vi "f_main_2014.vi"() -> ()   [LabVIEW 2014]
uses:
  <vilib>/Platform/TimedLoop/XDataNode/timing_clust.ctl
  <vilib>/Platform/TimedLoop/XDataNode/nitl_modes.ctl
  <vilib>/Platform/TimedLoop/XDataNode/wakeup.ctl
  <vilib>/rvi/Emulation/niFpgaGetClockAttributes.vi
  <vilib>/rvi/Emulation/niFpgaSctlEmulationGetInTimedLoop.vi
  <vilib>/rvi/Emulation/niFpgaEmulationReportErrorSimple.vi
  <vilib>/rvi/Emulation/niFpgaProcessEmulError.vi
  <vilib>/rvi/eio/common/nirviEmuTemplateMethod_errors.vi
  <vilib>/rvi/occurrence/nirviWaitOnOccurrenceBase.vi
  <vilib>/rvi/Emulation/niFpgaCriticalErrorInLSC.vi
  Instance           4 21Saved   f_main(DMA)85 .vi
  Instance           5 21Saved   f_main(DMA)85 .vi
  Instance           6 21Saved   f_main(DMA)85 .vi
  <vilib>/rvi/Memory/Memory_Emulation/nirvimemoryFastEmulation.vi
  <vilib>/rvi/Memory/Memory_Emulation/nirvimemoryEmulation.vi
  <vilib>/rvi/Emulation/niFpgaEmulationIsFPGAContextNoSignature.vi
  <vilib>/rvi/DataTransferAndStorage/Container/Common/niFpgaContainerGetUniqueNameForEmu.vi
  <vilib>/rvi/errors/nirviReportUnexpectedCaseInternalError (U32).vi
  <vilib>/rvi/interface/RandomDataEmulation/niFpgaRandomDataHandleErrors.vi
  Instance           2 21Saved   f_main(DMA)85 .vi
  Instance           3 21Saved   f_main(DMA)85 .vi
  <vilib>/eio/EIONode/EIONode.xnode
  <vilib>/Platform/TimedLoop/XDataNode/XDataNode.xnode
  <vilib>/rvi/DataTransferAndStorage/Container/XNode/niFpgaContainer.xnode
  <vilib>/rvi/interface/RandomDataEmulation/nirviRandomDataFpgaReadWriteTemplate.vi
  <vilib>/Platform/TimedLoop/XDataNode/XDNodeRunTimeDep.lvlib
panel:
  out "SampleTrigger3":u32
  out "SampleTrigger2":u32
  out "SampleTrigger1":u32
  out "SampleTrigger0":u32
  out "C3DIGIN":bool
  out "C2DIGIN":bool
  out "C0DIGIN":bool
  out "C1DIGIN":bool
  out "C3ADDREnable":bool
  out "C3Auswahl":bool
  out "C3ADDR3":bool
  out "C3ADDR2":bool
  out "C3ADDR1":bool
  out "C3ADDR0":bool
  out "C2ADDREnable":bool
  out "C2Auswahl":bool
  out "C2ADDR3":bool
  out "C2ADDR2":bool
  out "C2ADDR1":bool
  out "C2ADDR0":bool
  out "C1ADDREnable":bool
  out "C1Auswahl":bool
  out "C1ADDR3":bool
  out "C1ADDR2":bool
  out "C1ADDR1":bool
  out "C1ADDR0":bool
  in  "Test":bool
  in  "Timeout(in Ticks)":u32=4294967295
  out "cancel":bool
  out "Timeout":bool
  out "Sprung1":bool
  out "Sprung0":bool
  out "Fifo-Fehler":bool
  out "in\nReady":bool
  out "ScanID":u32
  in  "ADCRead":bool
  in  "read_count":u32
  out "C0ADDREnable":bool
  out "C0Auswahl":bool
  out "C0ADDR3":bool
  out "C0ADDR2":bool
  out "C0ADDR1":bool
  out "C0ADDR0":bool
  in  "SPIWrite":bool
  in  "Serial Data Out":bool[](array[boolean])=[FALSE, FALSE, FALSE, FALSE, FALSE, FALSE, FALSE, FALSE, FALSE, FALSE, FALSE, FALSE, FALSE, FALSE, FALSE, FALSE, FALSE, FALSE, FALSE, FALSE, FALSE, FALSE, FALSE, FALSE, FALSE, FALSE, FALSE, FALSE, FALSE, FALSE, FALSE, FALSE]
  in  "nbit":u8=16
  out "HIREF":bool
  out "SYNC":bool
  out "RESET":bool
  out "RLY2":bool
  out "RLY1":bool
  # "seriell Schreiben"
  # "seriell Lesen"
  # "Filter"
  # "Addressierung"
  # "sontiges"
  # "Kalibrierung"
  # "Triggerlines"
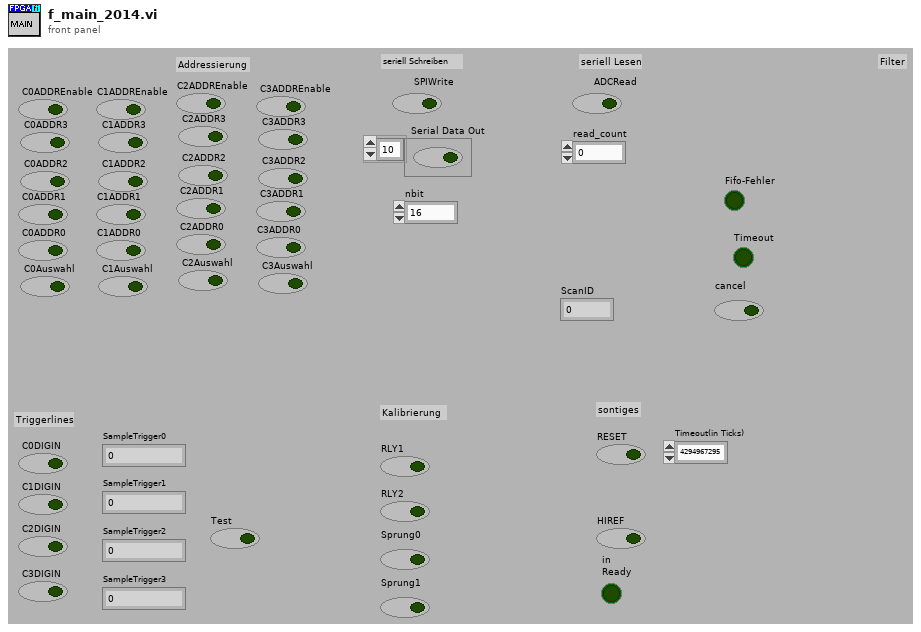
[diagram p1: front panel]
types:
  T1 = cluster{"occurrence":refnum<k4>, "occurrence":refnum<k4>, "occurrence":refnum<k4>, "occurrence":refnum<k4>}
  T2 = typedef "XDNodeRunTimeDep.lvlib/timing_clust.ctl" = cluster{"Expected End [f-1]":u64, "Actual End [f-1]":u64, "Finished Late? [f-1]":bool, "Expected End [i-1]":u64, "Actual End [i-1]":u64, "Finished Late? [i-1]":bool, "Expected Start [i]":u64, "Actual Start [i]":u64, "Expected Start [f]":u64, "Actual Start [f]":u64, "Source Name":string, "Structure Name":string, "Period":i64, "Deadline":i64, "Offset":i64, "Start":i64, "Priority":i32, "Timeout":i32, "Mode":T3, "Wakeup Reason":T4, "Error":errorcluster, "Source Type":string, "Secondary Source Type":string, "Global End Time":u64, "Global Start Time":u64, "Frame Duration":u64, "Iteration Duration":u64, "Assigned CPU":i32, "I/O Scan Engine Mode":u32}
  T3 = typedef "XDNodeRunTimeDep.lvlib/nitl_modes.ctl" = enum32{"No Change", "Process missed periods, maintain original phase", "Discard missed periods, maintain original phase", "Process missed periods, ignore original phase", "Discard missed periods, ignore original phase"}
  T4 = typedef "XDNodeRunTimeDep.lvlib/wakeup.ctl" = enum32{"Normal", "Aborted", "Asynchronous wakeup", "Timing source error", "Timed loop error", "Timeout"}
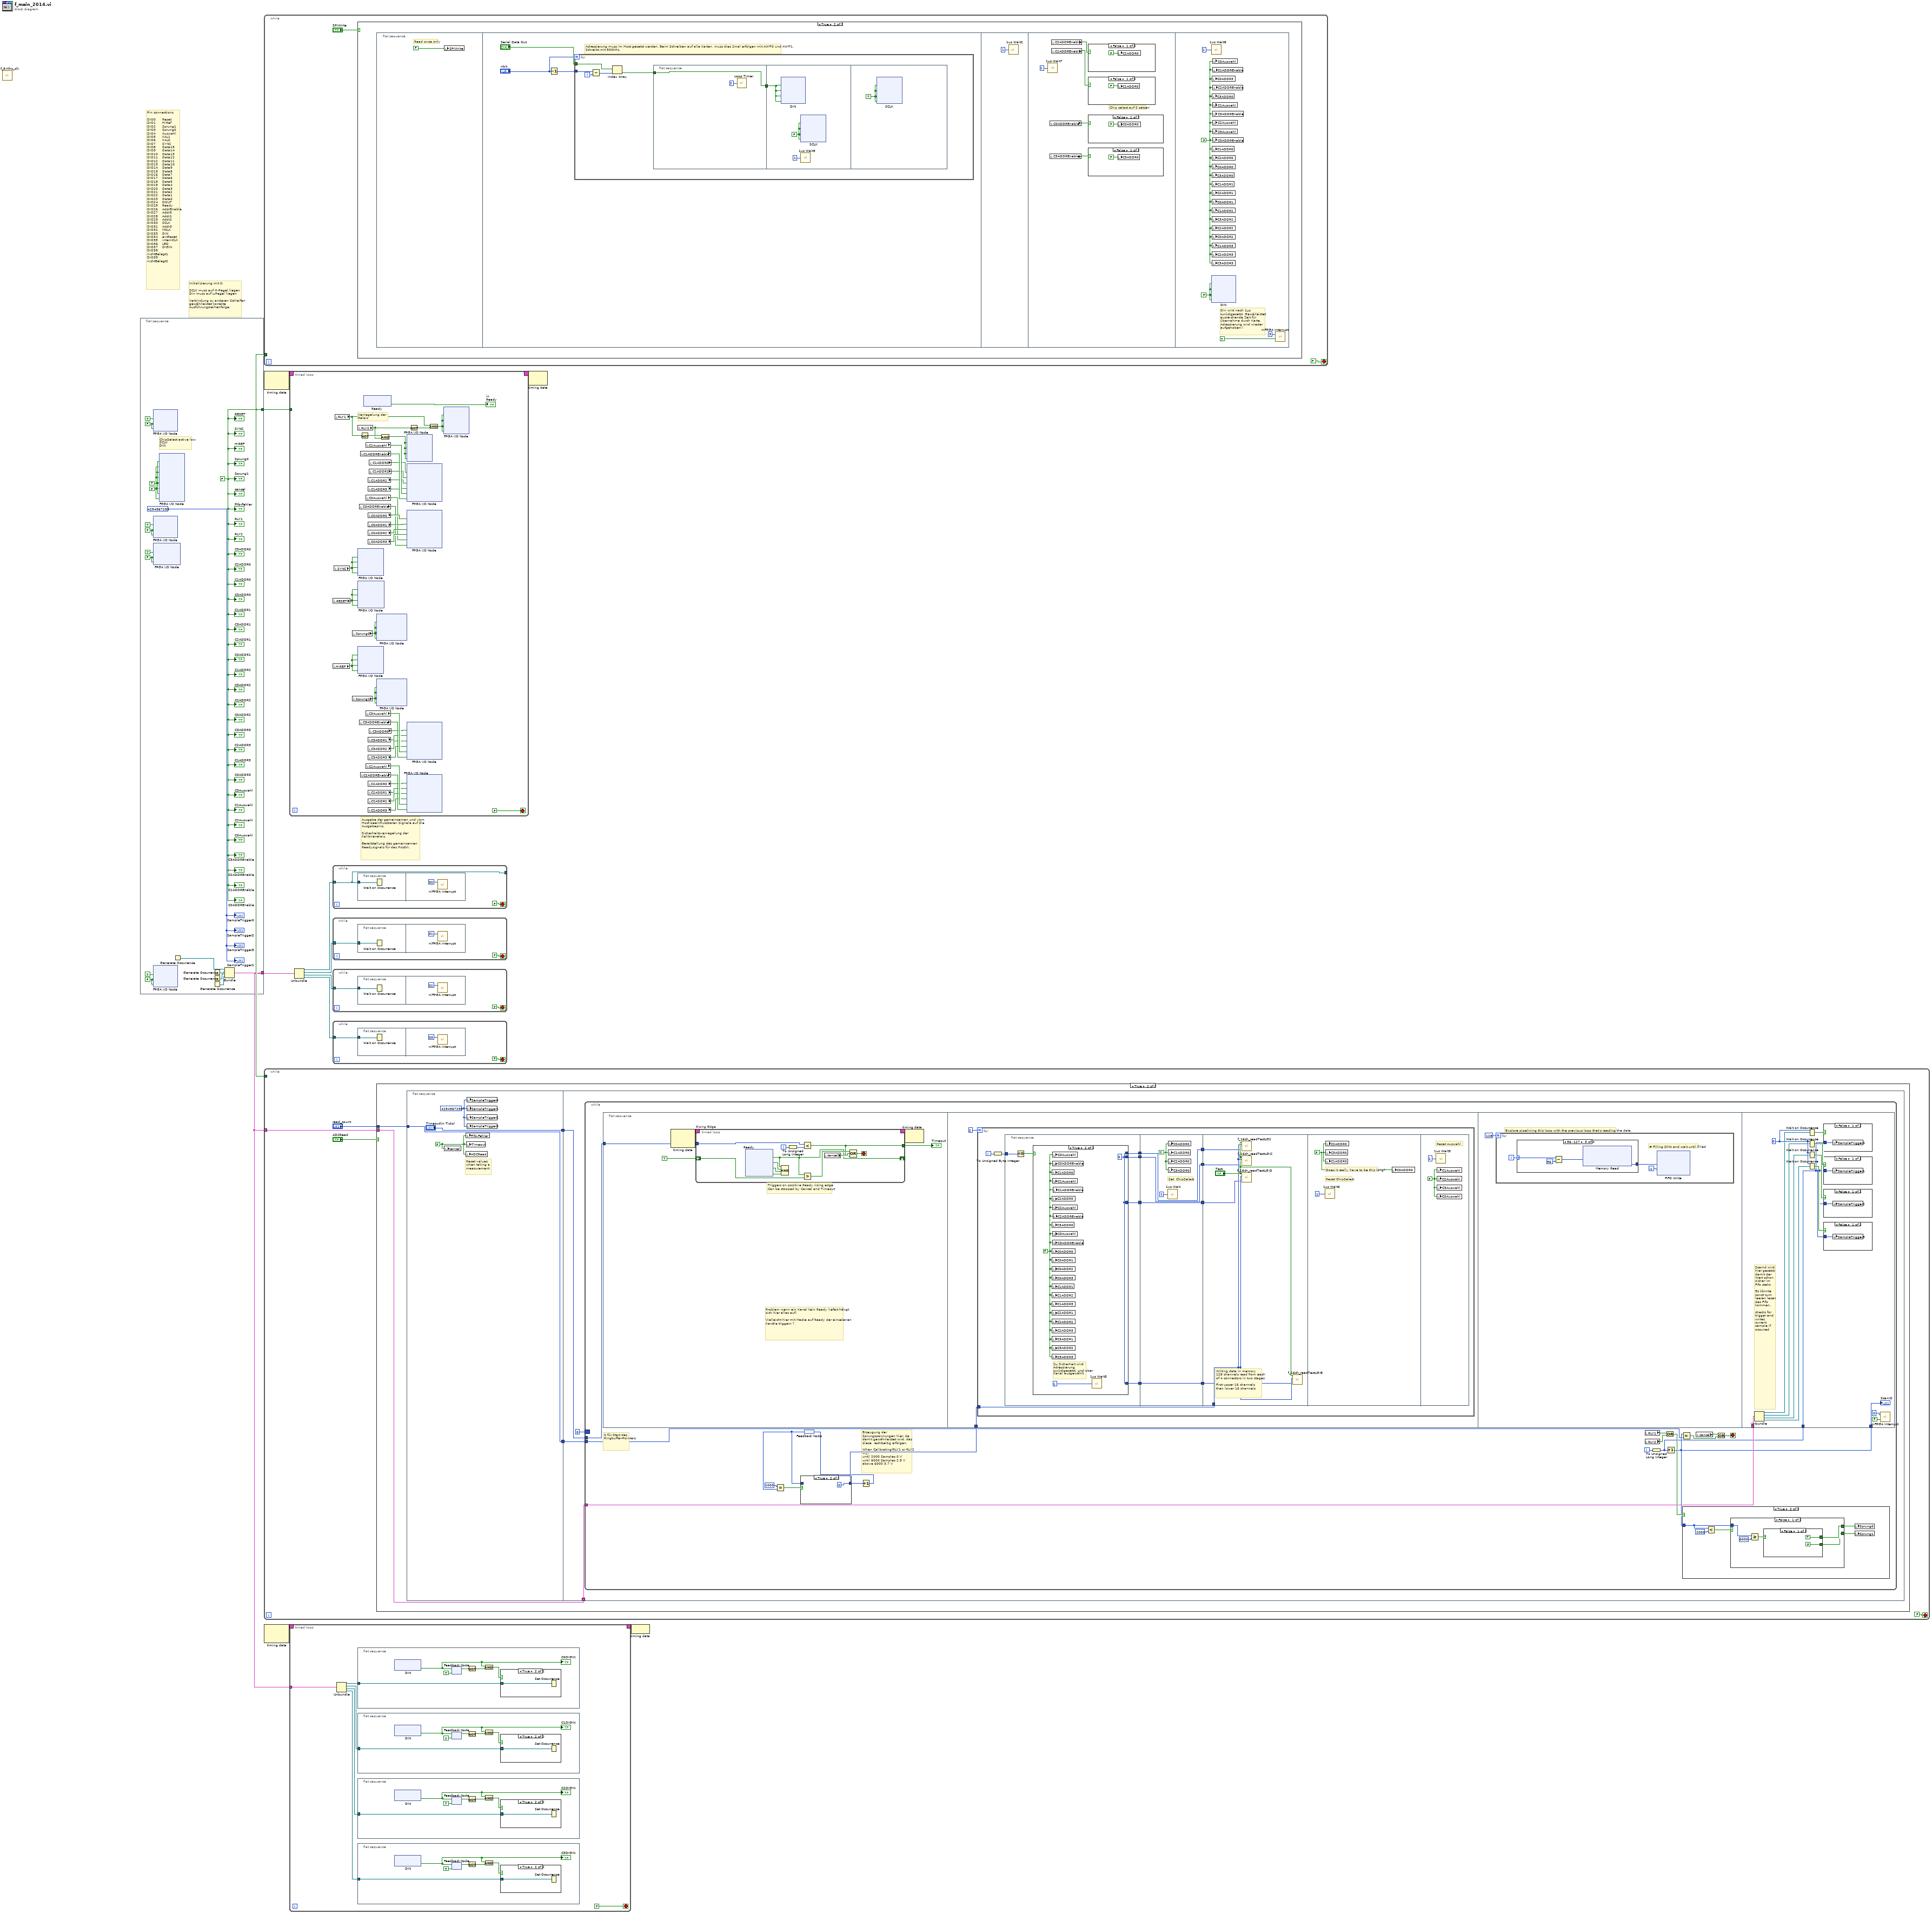
[diagram p0: block diagram]
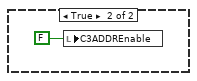
[diagram p7: hidden frame]
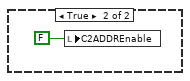
[diagram p8: hidden frame]
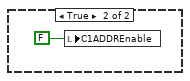
[diagram p9: hidden frame]
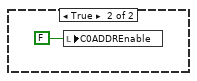
[diagram p10: hidden frame]
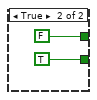
[diagram p14: hidden frame]
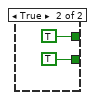
[diagram p15: hidden frame]
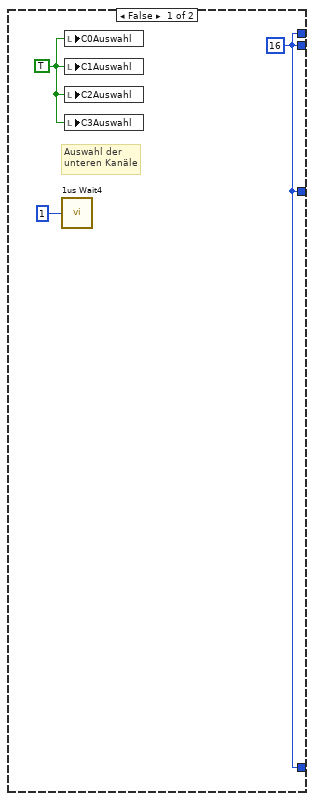
[diagram p16: hidden frame]
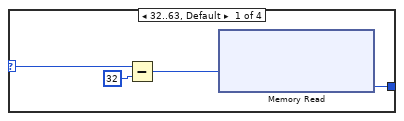
[diagram p17: hidden frame]
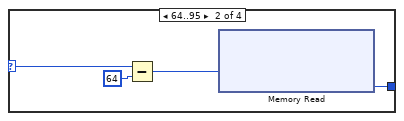
[diagram p18: hidden frame]
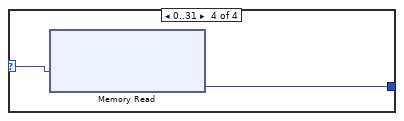
[diagram p19: hidden frame]
diagram:
  # "Pin connections\n\nDIO0      Reset\nDIO1      HiRef\nDIO2      Sprung1\nDIO3      Sprung0\nDIO4      Auswahl\nDIO5      KAL1\nDIO6      KAL0\nDIO7      SYNC\nDIO8      Data15\nDIO9      Data14\nDIO10    Data13\nDIO11    Data12\nDIO12    Data11\nDIO13    Data10\nDIO14    Data9\nDIO15    Data8\nDIO16    Data7\nDIO17    Data6\nDIO18    Data5\nDIO19    Data4\nDIO20    Data3\nDIO21    Data2\nDIO22    Data1\nDIO23    Data0\nDIO24    DOUT\nDIO25    Ready\nDIO26    AddrEnable\nDIO27    Addr3\nDIO28    Addr1\nDIO29    Addr2\nDIO30    SCLK\nDIO31    Addr0\nDIO32    MCLK\nDIO33    DIN\nDIO34    extReset\nDIO35    internCLK\nDIO36    LED\nDIO37    DIGIN\nDIO38    nichtBelegt1\nDIO39    nichtBelegt2"
  # "Initialisierung mit 0;\n\nSCLK muss auf H-Pegel liegen\nDin muss auf L-Pegel liegen\n\nVerbindung zu anderen Schleifen gewährleistet korrekte Ausführungsreihenfolge."
  # "Ausgabe der gemeinsamen und vom Host beeinflussbaren Signale auf die Ausgabepins. \n\nSicherheitsverriegelung der Kalibrierrelais.\n\nBereitstellung des gemeinsamen Readysignals für das HostVI."
  n1 = call "f_5-Mhz_clk.vi"() -> ()  [unwired: 1 out]
  n2 = flat-sequence {
    tunnel: [w23] -> w8
    tunnel: [w11] -> w1
    frame #0 {
      w16 = u32 4294967295 ("SampleTrigger0")
      w19 = FALSE
      w21 = FALSE
      w24 = FALSE
      w26 = FALSE
      w23 = FALSE
      w17 = FALSE ("Digital Data")
      w18 = TRUE ("Digital Data")
      # "ChipSelect active low\nSCLK\nDIN"
      n3 = xnode "FPGA I/O Node"("C1LED"=TRUE, "C1nb1"=w24, "C1nb2"=w24) -> ()  [unwired: 3 in, 3 out]
      n4 = xnode "FPGA I/O Node"("C3LED"=TRUE, "C3nb1"=w19, "C3nb2"=w19) -> ()  [unwired: 3 in, 3 out]
      n5 = xnode "FPGA I/O Node"("C0LED"=TRUE, "C0DIGIN"=w26, "C0nb2"=w26) -> ()  [unwired: 3 in, 3 out]
      n6 = xnode "FPGA I/O Node"("C2LED"=TRUE, "C2nb1"=w21, "C2nb2"=w21) -> ()  [unwired: 3 in, 3 out]
      n7 = xnode "FPGA I/O Node"("C0SCLK"=w18, "C0DIN"=w17, "C1SCLK"=w18, "C1DIN"=w17, "C2SCLK"=w18, "C2DIN"=w17, "C3SCLK"=w18, "C3DIN"=w17) -> ()  [unwired: 8 in, 8 out]
      n8 = Generate Occurrence() -> (w14:refnum<k4>)
      n9 = Generate Occurrence() -> (w15:refnum<k4>)
      n10 = Generate Occurrence() -> (w12:refnum<k4>)
      n11 = Generate Occurrence() -> (w13:refnum<k4>)
      n12 = Bundle("occurrence"=w14, "occurrence"=w15, "occurrence"=w12, "occurrence"=w13) -> (w11:T1)  [unwired: 1 in]
      "C0ADDR0" <- w23
      "C0ADDR1" <- w23
      "C0ADDR2" <- w23
      "C0ADDR3" <- w23
      "C0Auswahl" <- w23
      "C0ADDREnable" <- w23
      "RESET" <- w23
      "SYNC" <- w23
      "HIREF" <- w23
      "Sprung1" <- w23
      "Sprung0" <- w23
      "RLY1" <- w23
      "RLY2" <- w23
      "Fifo-Fehler" <- w23
      "cancel" <- w23
      "C1ADDR0" <- w23
      "C1ADDR1" <- w23
      "C1ADDR2" <- w23
      "C1ADDR3" <- w23
      "C1Auswahl" <- w23
      "C1ADDREnable" <- w23
      "C2ADDR0" <- w23
      "C2ADDR1" <- w23
      "C2ADDR2" <- w23
      "C2ADDR3" <- w23
      "C2Auswahl" <- w23
      "C2ADDREnable" <- w23
      "C3ADDR0" <- w23
      "C3ADDR1" <- w23
      "C3ADDR2" <- w23
      "C3ADDR3" <- w23
      "C3Auswahl" <- w23
      "C3ADDREnable" <- w23
      "SampleTrigger2" <- w16
      "SampleTrigger3" <- w16
      "SampleTrigger1" <- w16
      "SampleTrigger0" <- w16
    }
  }
  n13 = while {
    tunnel: w8 -> [_]
    stop <- FALSE stop-if-true
    n14 = case shown="True" "SPIWrite" {
      frame False {
      }
      frame True {
        n15 = flat-sequence {
          frame #0 {
            # "Read once only"
            n16 = local write "SPIWrite"(FALSE) -> ()
          }
          frame #1 {
            # "Adressierung muss im Host gesetzt werden. Beim Schreiben auf alle Karten, muss dies 2mal erfolgen mit AW=0 und AW=1.\nSchreibt mit 500kHz."
            n17 = Decrement(x="nbit") -> (x-1=w33:u8)
            n18 = for {
              N: "nbit" -> [_]
              tunnel: "Serial Data Out" -> [w37]
              tunnel: w33 -> [w39]
              i -> [w38]
              n19 = Subtract(x=w39, y=w38) -> (x-y=w36:i32)
              n20 = Index Array(array=w37, index=w36) -> (element=w35:bool)
              n21 = flat-sequence {
                tunnel: w35 -> [w41]
                tunnel: [w41] -> w34
                tunnel: w34 -> [w42]
                frame #0 {
                  n22 = call "Loop Timer"("Count(uSec)"=u32 2) -> ()  [unwired: 1 out]
                }
                frame #1 {
                  w43 = FALSE ("Digital Data")
                  n23 = xnode "DIN"("C0DIN"=w42, "C1DIN"=w42, "C2DIN"=w42, "C3DIN"=w42) -> ()  [unwired: 4 in, 4 out]
                  n24 = xnode "SCLK"("C0SCLK"=w43, "C1SCLK"=w43, "C2SCLK"=w43, "C3SCLK"=w43) -> ()  [unwired: 4 in, 4 out]
                  n25 = call "1us Wait5"("Count(uSec)"=u8 1) -> ()  [unwired: 1 out]
                }
                frame #2 {
                  w45 = TRUE ("Digital Data")
                  n26 = xnode "SCLK"("C0SCLK"=w45, "C1SCLK"=w45, "C2SCLK"=w45, "C3SCLK"=w45) -> ()  [unwired: 4 in, 4 out]
                }
              }
            }
          }
          frame #2 {
            n27 = call "1us Wait2"("Count(uSec)"=u8 1) -> ()  [unwired: 1 out]
          }
          frame #3 {
            # "Chip select auf 0 setzen"
            n28 = call "1us Wait7"("Count(uSec)"=u8 1) -> ()  [unwired: 1 out]
            n29 = local read "C0ADDREnable"() -> (w51:bool)
            n30 = local read "C3ADDREnable"() -> (w48:bool)
            n31 = local read "C2ADDREnable"() -> (w49:bool)
            n32 = local read "C1ADDREnable"() -> (w50:bool)
            n33 = case shown="False" w49 {
              frame False {
                n34 = local write "C2ADDR0"(FALSE ("Digital Data")) -> ()
              }
              frame True {
                n35 = local write "C2ADDREnable"(FALSE ("Digital Data")) -> ()
              }
            }
            n36 = case shown="False" w50 {
              frame False {
                n37 = local write "C1ADDR0"(FALSE ("Digital Data")) -> ()
              }
              frame True {
                n38 = local write "C1ADDREnable"(FALSE ("Digital Data")) -> ()
              }
            }
            n39 = case shown="False" w51 {
              frame False {
                n40 = local write "C0ADDR0"(FALSE ("Digital Data")) -> ()
              }
              frame True {
                n41 = local write "C0ADDREnable"(FALSE ("Digital Data")) -> ()
              }
            }
            n42 = case shown="False" w48 {
              frame False {
                n43 = local write "C3ADDR0"(FALSE ("Digital Data")) -> ()
              }
              frame True {
                n44 = local write "C3ADDREnable"(FALSE ("Digital Data")) -> ()
              }
            }
          }
          frame #4 {
            w62 = FALSE ("Digital Data")
            w60 = FALSE ("Digital Data")
            # "Din wird nach 1µs zurückgesetzt. Gewärleistet ausreichende Zeit für übernahme durch Karte.\nAdressierung wird wieder aufgehoben!!"
            n45 = call "1us Wait8"("Count(uSec)"=u8 1) -> ()  [unwired: 1 out]
            n46 = xnode "DIN"("C0DIN"=w60, "C1DIN"=w60, "C2DIN"=w60, "C3DIN"=w60) -> ()  [unwired: 4 in, 4 out]
            n47 = local write "C0ADDR3"(w62) -> ()
            n48 = local write "C3ADDR0"(w62) -> ()
            n49 = local write "C1ADDR0"(w62) -> ()
            n50 = local write "C2ADDR0"(w62) -> ()
            n51 = local write "C0ADDR0"(w62) -> ()
            n52 = local write "C3ADDR0"(w62) -> ()
            n53 = local write "C1ADDR1"(w62) -> ()
            n54 = local write "C2ADDR1"(w62) -> ()
            n55 = local write "C0ADDR1"(w62) -> ()
            n56 = local write "C1ADDR2"(w62) -> ()
            n57 = local write "C3ADDR2"(w62) -> ()
            n58 = local write "C2ADDR2"(w62) -> ()
            n59 = local write "C0ADDR2"(w62) -> ()
            n60 = local write "C1ADDR3"(w62) -> ()
            n61 = local write "C2ADDR3"(w62) -> ()
            n62 = local write "C3ADDR3"(w62) -> ()
            n63 = local write "C0Auswahl"(w62) -> ()
            n64 = local write "C1Auswahl"(w62) -> ()
            n65 = local write "C3ADDREnable"(w62) -> ()
            n66 = local write "C2Auswahl"(w62) -> ()
            n67 = local write "C3Auswahl"(w62) -> ()
            n68 = local write "C0ADDREnable"(w62) -> ()
            n69 = local write "C1ADDREnable"(w62) -> ()
            n70 = local write "C2ADDREnable"(w62) -> ()
            n71 = call <vilib>:"niFPGA Interrupt.vi"("Wait Until Cleared (F)"=TRUE ("Wait Until Cleared"), "IRQ Number (0)"=u8 3 ("IRQ Bit (0-31)")) -> ()  [unwired: 1 in]
          }
        }
      }
    }
  }
  n72 = node-c288() -> (w9:T2)  [unwired: 2 out]
  n73 = while {
    tunnel: w8 -> [_]
    tunnel: w1 -> [w65]
    stop <- FALSE stop-if-true
    n74 = case shown="True" "ADCRead" {
      tunnel: "read_count" -> [_ w70]
      tunnel: w65 -> [_ w69]
      frame False {
      }
      frame True {
        n75 = flat-sequence {
          tunnel: ["Timeout(in Ticks)"] -> w72
          tunnel: w70 -> [w74]
          tunnel: [w74] -> w71
          tunnel: w72 -> [w80]
          tunnel: w71 -> [w79]
          tunnel: w69 -> [w77]
          frame #0 {
            w73 = u32 4294967295 ("SampleTrigger1")
            w75 = FALSE
            # "Reset values when taking a measurement"
            n76 = local write "cancel"(w75) -> ()
            n77 = local write "Fifo-Fehler"(w75) -> ()
            n78 = local write "ADCRead"(w75) -> ()
            n79 = local write "Timeout"(w75) -> ()
            n80 = local write "SampleTrigger0"(w73) -> ()
            n81 = local write "SampleTrigger1"(w73) -> ()
            n82 = local write "SampleTrigger2"(w73) -> ()
            n83 = local write "SampleTrigger3"(w73) -> ()
          }
          frame #1 {
            n84 = while {
              tunnel: w80 -> [w92]
              tunnel: w79 -> [w84]
              border: u16 0 -> [_]
              tunnel: w77 -> [w82]
              i -> [w97]
              stop <- w93 stop-if-true
              # "0 für Start des Ringbuffer-Pointers"
              # "Erzeugung der Sprungspannungen hier, da damit gewährleistet wird, das diese  rechtzeitig erfolgen.\n\nWhen Calibrating(RLY1 or RLY2 =1) \nuntil 2000 Samples 0 V\nuntil 6000 Samples 2.5 V\nabove 6000 3.7 V"
              n85 = flat-sequence {
                tunnel: w92 -> [w119]
                tunnel: w89 -> [w138]
                tunnel: w85 -> [w209]
                tunnel: w82 -> [w206]
                tunnel: w81 -> [w200]
                frame #0 {
                  # "Triggers on positive Ready rising edge\nCan be stooped by Cancel and Timeout"
                  # "Problem wenn ein Kanal kein Ready liefert hängt sich hier alles auf!\n\nVielleicht hier mit Maske auf Ready der einzelenen Kanäle triggern ?"
                  n86 = node-c288() -> (w116:T2)  [unwired: 2 out]
                  n87 = timed-loop "Rising Edge" {
                    tunnel: [w127] -> w118
                    tunnel: w119 -> [w126]
                    timing-out: [_] -> w117
                    timing: w116 -> [_]
                    shift-left: TRUE ("DIOInput") -> [w132]
                    shift-right: [w121] -> _
                    i -> [w131]
                    stop <- w128 stop-if-true
                    n88 = xnode "Ready"() -> ("C0Ready"=w121:bool, "C1Ready"=w124:bool, "C2Ready"=w123:bool, "C3Ready"=w122:bool)  [unwired: 4 in, 4 out]
                    n89 = Compound Arithmetic op=AND(w121, w124, w123, w122) -> ()  [unwired: 1 out]
                    n90 = To Unsigned Long Integer(number=w131) -> (unsigned 32bit integer=w125:u32)
                    n91 = Less?(x=w126, y=w125) -> (x < y?=w127:bool)
                    n92 = Greater?(x=w121, y=w132) -> (0:w130:bool)
                    n93 = local read "cancel"() -> (w129:bool)
                    n94 = Compound Arithmetic op=OR(w130, w129, w127) -> (w128:bool)
                  }
                  "Timeout" <- w118
                  n95 = node-c288(w117) -> ()  [unwired: 1 out]
                }
                frame #1 {
                  n96 = for {
                    N: u8 2 -> [_]
                    tunnel: w138 -> [w147]
                    i -> [w149]
                    n97 = To Unsigned Byte Integer(number=w149) -> (unsigned 8bit integer=w148:u8)
                    n98 = flat-sequence {
                      tunnel: w148 -> [w154]
                      tunnel: [w153] -> w145
                      tunnel: [w152] -> w144
                      tunnel: [w151] -> w142
                      tunnel: [w150] -> w140
                      tunnel: [w166] -> w146
                      tunnel: w145 -> [w166]
                      tunnel: w144 -> [w165]
                      tunnel: [w165] -> w143
                      tunnel: w142 -> [w164]
                      tunnel: [w164] -> w141
                      tunnel: w140 -> [w163]
                      tunnel: [w163] -> w139
                      tunnel: w147 -> [w173]
                      tunnel: w146 -> [w171]
                      tunnel: w143 -> [w170]
                      tunnel: w141 -> [w169]
                      tunnel: w139 -> [w168]
                      frame #0 {
                        n99 = Equal To 0?(x=w154) -> (x = 0?=w155:bool)
                        n100 = case shown="True" w155 {
                          tunnel: [w156 w159] -> w153
                          tunnel: [w156 w159] -> w152
                          tunnel: [w156 w159] -> w151
                          tunnel: [w156 w159] -> w150
                          frame False {
                            w156 = u32 16
                            w157 = TRUE ("Digital Data")
                            # "Auswahl der unteren Kanäle"
                            n101 = call "1us Wait4"("Count(uSec)"=u8 1) -> ()  [unwired: 1 out]
                            n102 = local write "C0Auswahl"(w157) -> ()
                            n103 = local write "C1Auswahl"(w157) -> ()
                            n104 = local write "C2Auswahl"(w157) -> ()
                            n105 = local write "C3Auswahl"(w157) -> ()
                          }
                          frame True {
                            w159 = u32 0
                            w160 = FALSE ("Digital Data")
                            # "Zu Sicherheit wird Adressierung zurückgesetzt, und ober Kanal ausgewählt"
                            n106 = local write "C1ADDR0"(w160) -> ()
                            n107 = local write "C2ADDR0"(w160) -> ()
                            n108 = local write "C3ADDR0"(w160) -> ()
                            n109 = local write "C0ADDR0"(w160) -> ()
                            n110 = local write "C0ADDR1"(w160) -> ()
                            n111 = local write "C0ADDR2"(w160) -> ()
                            n112 = local write "C0ADDR3"(w160) -> ()
                            n113 = local write "C1ADDR1"(w160) -> ()
                            n114 = local write "C1ADDR2"(w160) -> ()
                            n115 = local write "C1ADDR3"(w160) -> ()
                            n116 = local write "C2ADDR1"(w160) -> ()
                            n117 = local write "C2ADDR2"(w160) -> ()
                            n118 = local write "C2ADDR3"(w160) -> ()
                            n119 = local write "C3ADDR1"(w160) -> ()
                            n120 = local write "C3ADDR2"(w160) -> ()
                            n121 = local write "C3ADDR3"(w160) -> ()
                            n122 = local write "C0Auswahl"(w160) -> ()
                            n123 = local write "C0ADDREnable"(w160) -> ()
                            n124 = local write "C1Auswahl"(w160) -> ()
                            n125 = local write "C2Auswahl"(w160) -> ()
                            n126 = local write "C3Auswahl"(w160) -> ()
                            n127 = local write "C3ADDREnable"(w160) -> ()
                            n128 = local write "C1ADDREnable"(w160) -> ()
                            n129 = local write "C2ADDREnable"(w160) -> ()
                            n130 = call "1us Wait3"("Count(uSec)"=u8 1) -> ()  [unwired: 1 out]
                          }
                        }
                      }
                      frame #1 {
                        w162 = TRUE
                        # "Set  ChipSelect"
                        n131 = call "1us Wait"("Count(uSec)"=u8 1) -> ()  [unwired: 1 out]
                        n132 = local write "C0ADDR0"(w162) -> ()
                        n133 = local write "C1ADDR0"(w162) -> ()
                        n134 = local write "C2ADDR0"(w162) -> ()
                        n135 = local write "C3ADDR0"(w162) -> ()
                      }
                      frame #2 {
                        # "Writing data in memory\n128 channels read from each of 4 connectors in two stages\n\nFirst upper 16 channels\nthen lower 16 channels"
                        n136 = call "f_16ch_readTestLG2.vi"("StartIndex"=w171, "Address"=w173, "Test"="Test") -> ()  [unwired: 5 out]
                        n137 = call "f_16ch_readTestLG-C.vi"("StartIndex"=w168, "Address"=w173, "Test"="Test") -> ()  [unwired: 5 out]
                        n138 = call "f_16ch_readTestLG-D.vi"("StartIndex"=w169, "Address"=w173, "Test"="Test") -> ()  [unwired: 5 out]
                        n139 = call "f_16ch_readTestLG-B.vi"("StartIndex"=w170, "Address"=w173, "Test"="Test") -> ()  [unwired: 5 out]
                      }
                      frame #3 {
                        w174 = FALSE
                        # "Does it really have to be this long?"
                        # "Reset ChipSelect"
                        n140 = call "1us Wait6"("Count(uSec)"=u8 1) -> ()  [unwired: 1 out]
                        n141 = local write "C2ADDR0"(w174) -> ()
                        n142 = local write "C3ADDR0"(w174) -> ()
                        n143 = local write "C1ADDR0"(w174) -> ()
                        n144 = local write "C0ADDR0"(w174) -> ()
                      }
                      frame #4 {
                        w177 = FALSE
                        # "Reset Auswahl"
                        n145 = call "1us Wait9"("Count(uSec)"=u8 1) -> ()  [unwired: 1 out]
                        n146 = local write "C1Auswahl"(w177) -> ()
                        n147 = local write "C2Auswahl"(w177) -> ()
                        n148 = local write "C3Auswahl"(w177) -> ()
                        n149 = local write "C0Auswahl"(w177) -> ()
                      }
                    }
                  }
                }
                frame #2 {
                  # "Explore pipelining this loop with the previous loop that's reading the data."
                  n150 = for {
                    N: u8 128 -> [_]
                    i -> [w181]
                    # "# Filling DMA and wait until filled"
                    n151 = case shown="96..127" w181 {
                      selector: w181 -> [w184 w187 w192 w194]
                      tunnel: [w185 w189 w193 w195] -> w180
                      frame 32..63, Default {
                        n152 = Subtract(x=w184, y=32) -> (x-y=w183:i32)
                        n153 = xnode ("Memory Read")("Address"=w183) -> ("Data"=w185:i16)  [unwired: 1 in, 1 out]
                      }
                      frame 64..95 {
                        n154 = Subtract(x=w187, y=64) -> (x-y=w188:i32)
                        n155 = xnode ("Memory Read")("Address"=w188) -> ("Data"=w189:i16)  [unwired: 1 in, 1 out]
                      }
                      frame 96..127 {
                        n156 = Subtract(x=w192, y=96) -> (x-y=w191:i32)
                        n157 = xnode ("Memory Read")("Address"=w191) -> ("Data"=w193:i16)  [unwired: 1 in, 1 out]
                      }
                      frame 0..31 {
                        n158 = xnode ("Memory Read")("Address"=w194) -> ("Data"=w195:i16)  [unwired: 1 in, 1 out]
                      }
                    }
                    n159 = xnode ("FIFO Write")("Element"=w180, "Timeout"=i8 -1) -> ()  [unwired: 1 in, 2 out]
                  }
                }
                frame #3 {
                  w202 = 0 ("ms timeout (-1)")
                  # "ScanId wird hier gesetzt damit der Wert schon sicher im Fifo steht.\n\nEs könnte sonst zum leeren lesen des Fifo kommen. \n\nchecks for trigger and writes current sample if occurred"
                  n160 = Unbundle(w206) -> ("occurrence"=w199:refnum<k4>, "occurrence"=w198:refnum<k4>, "occurrence"=w197:refnum<k4>, "occurrence"=w196:refnum<k4>)
                  n161 = Wait on Occurrence(2:w199, 3:w202) -> (0:w205:bool)  [unwired: 1 in]
                  n162 = Wait on Occurrence(2:w198, 3:w202) -> (0:w204:bool)  [unwired: 1 in]
                  n163 = Wait on Occurrence(2:w197, 3:w202) -> (0:w201:bool)  [unwired: 1 in]
                  n164 = Wait on Occurrence(2:w196, 3:w202) -> (0:w203:bool)  [unwired: 1 in]
                  n165 = case shown="False" w205 {
                    tunnel: w200 -> [w213 _]
                    frame False {
                      n166 = local write "SampleTrigger0"(w213) -> ()
                    }
                    frame True {
                    }
                  }
                  n167 = case shown="False" w204 {
                    tunnel: w200 -> [w212 _]
                    frame False {
                      n168 = local write "SampleTrigger1"(w212) -> ()
                    }
                    frame True {
                    }
                  }
                  n169 = case shown="False" w201 {
                    tunnel: w200 -> [w210 _]
                    frame False {
                      n170 = local write "SampleTrigger2"(w210) -> ()
                    }
                    frame True {
                    }
                  }
                  n171 = case shown="False" w203 {
                    tunnel: w200 -> [w211 _]
                    frame False {
                      n172 = local write "SampleTrigger3"(w211) -> ()
                    }
                    frame True {
                    }
                  }
                  n173 = call <vilib>:"niFPGA Interrupt.vi"("Wait Until Cleared (F)"=FALSE ("Wait Until Cleared"), "IRQ Number (0)"=u8 0) -> ()  [unwired: 1 in]
                  "ScanID" <- w209
                }
              }
              n174 = feedback #1() -> (w88:u16)
              n175 = Equal?(x=u16 1000, y=w88) -> (x = y?=w90:bool)
              n176 = case shown="True" w90 {
                tunnel: [w98 u16 0] -> w89
                tunnel: w88 -> [w98 _]
                frame False {
                }
                frame True {
                }
              }
              n177 = Increment(x=w89) -> (x+1=w87:u16)
              n178 = feedback-in #1(w87) -> ()
              n179 = local read "RLY1"() -> (w95:bool)
              n180 = local read "RLY2"() -> (w94:bool)
              n181 = To Unsigned Long Integer(number=w97) -> (unsigned 32bit integer=w81:u32)
              n182 = Or(x=w95, y=w94) -> (x .or. y?=w96:bool)
              n183 = Increment(x=w81) -> (x+1=w85:u32)
              n184 = Equal?(x=w85, y=w84) -> (x = y?=w91:bool)
              n185 = case shown="True" w96 {
                tunnel: w85 -> [_ w102]
                frame False {
                }
                frame True {
                  n186 = Less?(x=w102, y=u16 2000) -> (x < y?=w103:bool)
                  n187 = case shown="False" w103 {
                    tunnel: w102 -> [w108 _]
                    tunnel: [w106 TRUE] -> w101
                    tunnel: [w105 TRUE] -> w100
                    frame False {
                      n188 = Greater Or Equal?(x=w108, y=u16 6000) -> (x >= y?=w107:bool)
                      n189 = case shown="False" w107 {
                        tunnel: [TRUE FALSE] -> w106
                        tunnel: [FALSE TRUE] -> w105
                        frame False {
                        }
                        frame True {
                        }
                      }
                    }
                    frame True {
                    }
                  }
                  n190 = local write "Sprung0"(w101) -> ()
                  n191 = local write "Sprung1"(w100) -> ()
                }
              }
              n192 = local read "cancel"() -> (w83:bool)
              n193 = Or(x=w83, y=w91) -> (x .or. y?=w93:bool)
            }
          }
        }
      }
    }
  }
  n194 = node-c288() -> (w3:T2)  [unwired: 2 in]
  n195 = timed-loop {
    timing-out: [_] -> w10
    timing: w9 -> [_]
    tunnel: w8 -> [_]
    stop <- FALSE stop-if-true
    # "Verriegelung der Relais"
    n196 = local read "HIREF"() -> (w242:bool)
    n197 = local read "RESET"() -> (w243:bool)
    n198 = local read "SYNC"() -> (w241:bool)
    n199 = local read "RLY1"() -> (w247:bool)
    n200 = local read "Sprung0"() -> (w240:bool)
    n201 = local read "Sprung1"() -> (w239:bool)
    n202 = xnode "FPGA I/O Node"("C0SYNC"=w241, "C1SYNC"=w241, "C2SYNC"=w241, "C3SYNC"=w241) -> ()  [unwired: 4 in, 4 out]
    n203 = xnode "FPGA I/O Node"("C0Reset"=w243, "C1Reset"=w243, "C2Reset"=w243, "C3Reset"=w243) -> ()  [unwired: 4 in, 4 out]
    n204 = xnode "FPGA I/O Node"("C0HiRef"=w242, "C1HiRef"=w242, "C2HiRef"=w242, "C3HiRef"=w242) -> ()  [unwired: 4 in, 4 out]
    n205 = local read "RLY2"() -> (w246:bool)
    n206 = local read "C0ADDREnable"() -> (w232:bool)
    n207 = local read "C3ADDREnable"() -> (w219:bool)
    n208 = Not(x=w247) -> (.not. x?=w249:bool)
    n209 = local read "C1ADDREnable"() -> (w231:bool)
    n210 = local read "C2ADDREnable"() -> (w225:bool)
    n211 = xnode "Ready"() -> ("C0Ready"=→"in\nReady":bool)  [unwired: 1 in, 1 out]
    n212 = local read "C1Auswahl"() -> (w230:bool)
    n213 = local read "C0Auswahl"() -> (w233:bool)
    n214 = local read "C3Auswahl"() -> (w218:bool)
    n215 = local read "C2Auswahl"() -> (w224:bool)
    n216 = local read "C1ADDR2"() -> (w227:bool)
    n217 = local read "C1ADDR3"() -> (w226:bool)
    n218 = local read "C0ADDR0"() -> (w237:bool)
    n219 = local read "C0ADDR1"() -> (w236:bool)
    n220 = local read "C0ADDR2"() -> (w235:bool)
    n221 = local read "C0ADDR3"() -> (w234:bool)
    n222 = local read "C3ADDR1"() -> (w215:bool)
    n223 = local read "C3ADDR2"() -> (w216:bool)
    n224 = local read "C3ADDR3"() -> (w217:bool)
    n225 = local read "C2ADDR0"() -> (w220:bool)
    n226 = local read "C2ADDR1"() -> (w221:bool)
    n227 = local read "C2ADDR2"() -> (w222:bool)
    n228 = local read "C2ADDR3"() -> (w223:bool)
    n229 = local read "C1ADDR0"() -> (w229:bool)
    n230 = local read "C1ADDR1"() -> (w228:bool)
    n231 = local read "C3ADDR0"() -> (w214:bool)
    n232 = xnode "FPGA I/O Node"("C0Sprung0"=w240, "C1Sprung0"=w240, "C2Sprung0"=w240, "C3Sprung0"=w240) -> ()  [unwired: 4 in, 4 out]
    n233 = xnode "FPGA I/O Node"("C0Sprung1"=w239, "C1Sprung1"=w239, "C2Sprung1"=w239, "C3Sprung1"=w239) -> ()  [unwired: 4 in, 4 out]
    n234 = And(x=w249, y=w246) -> (x .and. y?=w244:bool)
    n235 = xnode "FPGA I/O Node"("C0KAL1"=w244, "C1KAL1"=w244, "C2KAL1"=w244, "C3KAL1"=w244) -> ()  [unwired: 4 in, 4 out]
    n236 = xnode "FPGA I/O Node"("C1Addr0"=w229, "C1Addr1"=w228, "C1Addr2"=w227, "C1Addr3"=w226, "C1Auswahl"=w230, "C1AddrEnable"=w231) -> ()  [unwired: 6 in, 6 out]
    n237 = xnode "FPGA I/O Node"("C0Addr0"=w237, "C0Addr1"=w236, "C0Addr2"=w235, "C0Addr3"=w234, "C0Auswahl"=w233, "C0AddrEnable"=w232) -> ()  [unwired: 6 in, 6 out]
    n238 = xnode "FPGA I/O Node"("C3Addr0"=w214, "C3Addr1"=w215, "C3Addr2"=w216, "C3Addr3"=w217, "C3Auswahl"=w218, "C3AddrEnable"=w219) -> ()  [unwired: 6 in, 6 out]
    n239 = xnode "FPGA I/O Node"("C2Addr0"=w220, "C2Addr1"=w221, "C2Addr2"=w222, "C2Addr3"=w223, "C2Auswahl"=w224, "C2AddrEnable"=w225) -> ()  [unwired: 6 in, 6 out]
    n240 = Not(x=w246) -> (.not. x?=w248:bool)
    n241 = And(x=w247, y=w248) -> (x .and. y?=w238:bool)
    n242 = xnode "FPGA I/O Node"("C0KAL0"=w238, "C1KAL0"=w238, "C2KAL0"=w238, "C3KAL0"=w238) -> ()  [unwired: 4 in, 4 out]
  }
  n243 = timed-loop {
    timing: w3 -> [_]
    timing-out: [_] -> w2
    tunnel: w1 -> [w257]
    stop <- FALSE stop-if-true
    n244 = Unbundle(w257) -> ("occurrence"=w256:refnum<k4>, "occurrence"=w255:refnum<k4>, "occurrence"=w254:refnum<k4>, "occurrence"=w253:refnum<k4>)
    n245 = flat-sequence {
      tunnel: w256 -> [w269]
      frame #0 {
        n246 = xnode "DIN"() -> ("C0DIGIN"=w266:bool)  [unwired: 1 in, 1 out]
        "C0DIGIN" <- w266
        n247 = feedback #2(TRUE) -> (w267:bool)
        n248 = feedback-in #2(w266) -> ()
        n249 = Not(x=w267) -> (.not. x?=w271:bool)
        n250 = And(x=w266, y=w271) -> (x .and. y?=w270:bool)
        n251 = case shown="True" w270 {
          tunnel: w269 -> [_ w272]
          frame False {
          }
          frame True {
            n252 = Set Occurrence(w272) -> ()
          }
        }
      }
    }
    n253 = flat-sequence {
      tunnel: w255 -> [w264]
      frame #0 {
        n254 = xnode "DIN"() -> ("C1DIGIN"=w261:bool)  [unwired: 1 in, 1 out]
        "C1DIGIN" <- w261
        n255 = feedback-in #3(w261) -> ()
        n256 = feedback #3(TRUE) -> (w260:bool)
        n257 = Not(x=w260) -> (.not. x?=w263:bool)
        n258 = And(x=w261, y=w263) -> (x .and. y?=w259:bool)
        n259 = case shown="True" w259 {
          tunnel: w264 -> [_ w265]
          frame False {
          }
          frame True {
            n260 = Set Occurrence(w265) -> ()
          }
        }
      }
    }
    n261 = flat-sequence {
      tunnel: w254 -> [w278]
      frame #0 {
        n262 = xnode "DIN"() -> ("C2DIGIN"=w273:bool)  [unwired: 1 in, 1 out]
        "C2DIGIN" <- w273
        n263 = feedback #4(TRUE) -> (w274:bool)
        n264 = feedback-in #4(w273) -> ()
        n265 = Not(x=w274) -> (.not. x?=w276:bool)
        n266 = And(x=w273, y=w276) -> (x .and. y?=w277:bool)
        n267 = case shown="True" w277 {
          tunnel: w278 -> [_ w279]
          frame False {
          }
          frame True {
            n268 = Set Occurrence(w279) -> ()
          }
        }
      }
    }
    n269 = flat-sequence {
      tunnel: w253 -> [w285]
      frame #0 {
        n270 = xnode "DIN"() -> ("C3DIGIN"=w280:bool)  [unwired: 1 in, 1 out]
        "C3DIGIN" <- w280
        n271 = feedback #5(TRUE) -> (w281:bool)
        n272 = feedback-in #5(w280) -> ()
        n273 = Not(x=w281) -> (.not. x?=w283:bool)
        n274 = And(x=w280, y=w283) -> (x .and. y?=w284:bool)
        n275 = case shown="True" w284 {
          tunnel: w285 -> [_ w286]
          frame False {
          }
          frame True {
            n276 = Set Occurrence(w286) -> ()
          }
        }
      }
    }
  }
  n277 = Unbundle(w1) -> ("occurrence"=w6:refnum<k4>, "occurrence"=w4:refnum<k4>, "occurrence"=w5:refnum<k4>, "occurrence"=w7:refnum<k4>)
  n278 = while {
    tunnel: [w289] -> _
    tunnel: w6 -> [w289]
    stop <- FALSE stop-if-true
    n279 = flat-sequence {
      tunnel: w289 -> [w291]
      frame #0 {
        n280 = Wait on Occurrence(2:w291) -> ()  [unwired: 2 in, 1 out]
      }
      frame #1 {
        n281 = call <vilib>:"niFPGA Interrupt.vi"("IRQ Number (0)"=u8 30 ("IRQ Bit (0-31)")) -> ()  [unwired: 2 in]
      }
    }
  }
  n282 = while {
    tunnel: w4 -> [w293]
    stop <- FALSE stop-if-true
    n283 = flat-sequence {
      tunnel: w293 -> [w295]
      frame #0 {
        n284 = Wait on Occurrence(2:w295) -> ()  [unwired: 2 in, 1 out]
      }
      frame #1 {
        n285 = call <vilib>:"niFPGA Interrupt.vi"("IRQ Number (0)"=u8 31 ("IRQ Bit (0-31)")) -> ()  [unwired: 2 in]
      }
    }
  }
  n286 = while {
    tunnel: w5 -> [w297]
    stop <- FALSE stop-if-true
    n287 = flat-sequence {
      tunnel: w297 -> [w299]
      frame #0 {
        n288 = Wait on Occurrence(2:w299) -> ()  [unwired: 2 in, 1 out]
      }
      frame #1 {
        n289 = call <vilib>:"niFPGA Interrupt.vi"("IRQ Number (0)"=u8 32 ("IRQ Bit (0-31)")) -> ()  [unwired: 2 in]
      }
    }
  }
  n290 = while {
    tunnel: w7 -> [w301]
    stop <- FALSE stop-if-true
    n291 = flat-sequence {
      tunnel: w301 -> [w303]
      frame #0 {
        n292 = Wait on Occurrence(2:w303) -> ()  [unwired: 2 in, 1 out]
      }
      frame #1 {
        n293 = call <vilib>:"niFPGA Interrupt.vi"("IRQ Number (0)"=u8 33 ("IRQ Bit (0-31)")) -> ()  [unwired: 2 in]
      }
    }
  }
  n294 = node-c288(w10) -> ()  [unwired: 1 out]
  n295 = node-c288(w2) -> ()
